vi "Pre Launch Init.vi"(11 "SM140 Actor in":refnum<class "SM140 Actor.lvclass">) -> (0 "error out":errorcluster, 3 "SM140 Actor out":refnum<class "SM140 Actor.lvclass">)   [LabVIEW 2017, in "SM140.lvlib" / "SM140 Actor.lvclass"]
doc: "Sends a high priority message to it's self to notify the monitor that it's spawned. If it's in the runtime environment, this message is never sent, meaning the monitor will never spawn\n\nCopyright: MGI\nAuthored by: Derek Trepanier"
uses:
  SM140 Actor.lvclass
  SM140 Actor.lvclass/SM140 Actor.ctl
  Actor Monitor/Actor/Monitored Actor.lvclass
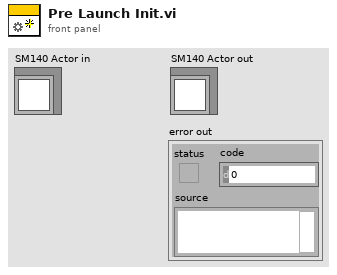
[diagram p1: front panel]
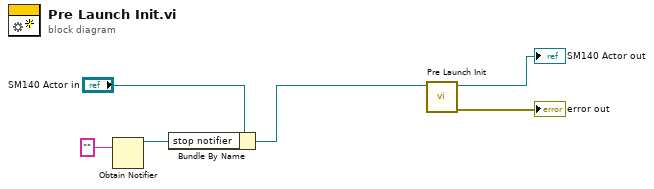
[diagram p0: block diagram]
diagram:
  n1 = Obtain Notifier(notification data type="") -> (notifier out=w3:refnum<notifier>)  [unwired: 3 in, 2 out]
  n2 = Bundle By Name(cluster="SM140 Actor in", "stop notifier"=w3) -> (w1:refnum<class "SM140 Actor.lvclass">)
  n3 = call-parent "Pre Launch Init.vi"("Monitored Actor in"=w1) -> ("error out"=→"error out":errorcluster, "Monitored Actor out"=→"SM140 Actor out":refnum<class "SM140 Actor.lvclass">)  [unwired: 9 in]
